vi "Ej 19 Display 7 seg.vi"() -> ()   [LabVIEW 2021]
panel:
  out "Unidades":bool
  out "Decenas":bool
  out "Centenas":bool
  in  "Selector":i32
  out "b":bool
  out "g":bool
  out "c":bool
  out "a":bool
  out "d":bool
  out "e":bool
  out "f":bool
  in  "stop":bool
  out "Unidades":dbl
  out "Decenas":dbl
  out "Centenas":dbl
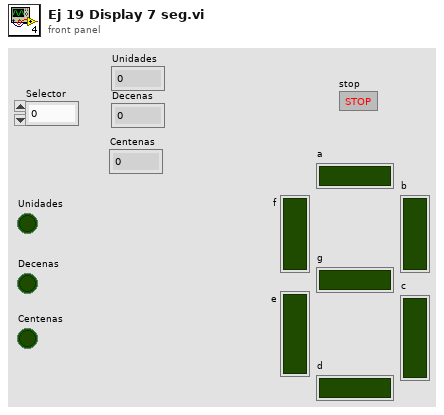
[diagram p1: front panel]
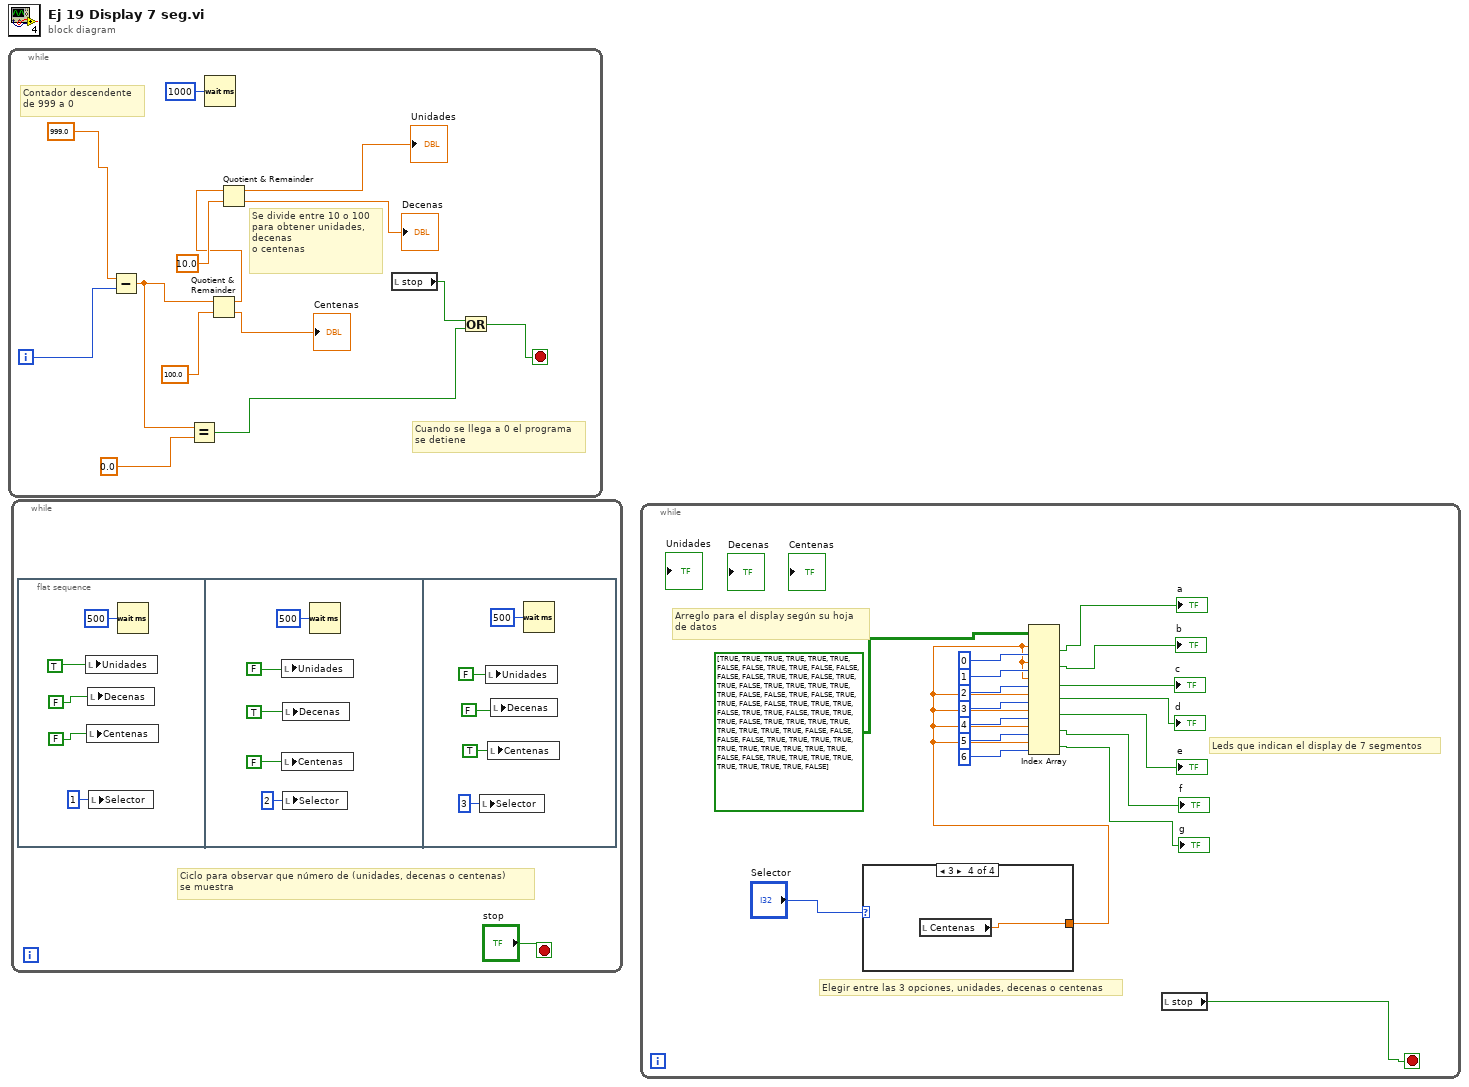
[diagram p0: block diagram]
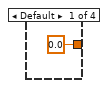
[diagram p2: hidden frame]
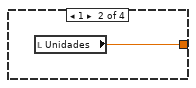
[diagram p3: hidden frame]
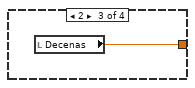
[diagram p4: hidden frame]
diagram:
  n1 = while {
    i -> [w2]
    stop <- w8 stop-if-true
    # "Cuando se llega a 0 el programa\nse detiene"
    # "Contador descendente\nde 999 a 0"
    # "Se divide entre 10 o 100 \npara obtener unidades, decenas\no centenas"
    n2 = Subtract(x=999.0, y=w2) -> (x-y=w1:dbl)
    n3 = Equal?(x=w1, y=0.0) -> (x = y?=w10:bool)
    n4 = Wait (ms)(milliseconds to wait=u32 1000) -> ()  [unwired: 1 out]
    n5 = Quotient & Remainder(x=w1, y=100.0) -> (x-y*floor(x/y)=w4:dbl, floor(x/y)=→"Centenas":dbl)
    n6 = Quotient & Remainder(x=w4, y=10.0) -> (x-y*floor(x/y)=→"Unidades":dbl, floor(x/y)=→"Decenas":dbl)
    n7 = local read "stop"() -> (w9:bool)
    n8 = Or(x=w9, y=w10) -> (x .or. y?=w8:bool)
  }
  n9 = while {
    stop <- "stop" stop-if-true
    # "Ciclo para observar que número de (unidades, decenas o centenas)\nse muestra"
    n10 = flat-sequence {
      frame #0 {
        n11 = local write "Unidades"(TRUE) -> ()
        n12 = local write "Centenas"(FALSE) -> ()
        n13 = local write "Decenas"(FALSE) -> ()
        n14 = local write "Selector"(1 ("Selector")) -> ()
        n15 = Wait (ms)(milliseconds to wait=u32 500) -> ()  [unwired: 1 out]
      }
      frame #1 {
        n16 = local write "Unidades"(FALSE) -> ()
        n17 = local write "Centenas"(FALSE) -> ()
        n18 = local write "Decenas"(TRUE) -> ()
        n19 = local write "Selector"(2 ("Selector")) -> ()
        n20 = Wait (ms)(milliseconds to wait=u32 500) -> ()  [unwired: 1 out]
      }
      frame #2 {
        n21 = local write "Selector"(3 ("Selector")) -> ()
        n22 = local write "Unidades"(FALSE) -> ()
        n23 = local write "Centenas"(TRUE) -> ()
        n24 = local write "Decenas"(FALSE) -> ()
        n25 = Wait (ms)(milliseconds to wait=u32 500) -> ()  [unwired: 1 out]
      }
    }
  }
  n26 = while {
    stop <- w38 stop-if-true
    # "Arreglo para el display según su hoja\nde datos"
    # "Leds que indican el display de 7 segmentos"
    # "Elegir entre las 3 opciones, unidades, decenas o centenas"
    n27 = case shown="3" "Selector" {
      tunnel: [0.0 ("Decenas") w50 w51 w52] -> w40
      frame Default {
      }
      frame 1 {
        n28 = local read "Unidades"() -> (w50:dbl)
      }
      frame 2 {
        n29 = local read "Decenas"() -> (w51:dbl)
      }
      frame 3 {
        n30 = local read "Centenas"() -> (w52:dbl)
      }
    }
    n31 = Index Array(array=bool[][] [[TRUE, TRUE, TRUE, TRUE, TRUE, TRUE, FALSE], [FALSE, TRUE, TRUE, FALSE, FALSE, FALSE, FALSE], [TRUE, TRUE, FALSE, TRUE, TRUE, FALSE, TRUE], [TRUE, TRUE, TRUE, TRUE, FALSE, FALSE, TRUE], [FALSE, TRUE, TRUE, FALSE, FALSE, TRUE, TRUE], [TRUE, FALSE, TRUE, TRUE, FALSE, TRUE, TRUE], [TRUE, FALSE, TRUE, TRUE, TRUE, TRUE, TRUE], [TRUE, TRUE, TRUE, FALSE, FALSE, FALSE, FALSE], [TRUE, TRUE, TRUE, TRUE, TRUE, TRUE, TRUE], [TRUE, TRUE, TRUE, FALSE, FALSE, TRUE, TRUE], [TRUE, TRUE, TRUE, TRUE, TRUE, TRUE, FALSE]], index (row) #1=w40, index (col) #1=0 ("disabled index (col)"), index (row) #2=w40, index (col) #2=1 ("index (col)"), index (row) #3=w40, index (col) #3=2 ("index (col)"), index (row) #4=w40, index (col) #4=3 ("index (col)"), index (row) #5=w40, index (col) #5=4 ("index (col)"), index (row) #6=w40, index (col) #6=5 ("index (col)"), index (row) #7=w40, index (col) #7=6 ("index (col)")) -> (element #1=→"a":bool, element #2=→"b":bool, element #3=→"c":bool, element #4=→"d":bool, element #5=→"e":bool, element #6=→"f":bool, element #7=→"g":bool)
    n32 = local read "stop"() -> (w38:bool)
  }
